vi "NI-DCPower Pulse Voltage Sequence T4.vi"() -> ()   [LabVIEW 2021, in "Main T4.lvlib"]
doc: "Demonstrates how to use the DCPower Pulse API to generate a Voltage Pulse Sequence. This example initializes a session, configures the Source Mode and the Output Function, configures the pulse parameters, initiates the pulse output sequence, and takes measurements."
uses:
  Main T4.lvlib
  DMM/controls/DMM Meas Type.ctl
  controls/Temp T4.ctl
  <instrlib>/niDCPower/nidcpower.llb/niDCPower Source Mode.ctl
  <instrlib>/niDCPower/nidcpower.llb/niDCPower Aperture Time Units.ctl
  <instrlib>/niDCPower/nidcpower.llb/niDCPower Output Function.ctl
  <instrlib>/niDCPower/nidcpower.llb/niDCPower Wait For Event - Event.ctl
  DMM/DMM T4.lvlib
panel:
  out "Cluster 2":T1={"Read?"=TRUE, "Temp"=0}
  in  "Cluster":T1={"Read?"=TRUE, "Temp"=0}
  in  "SMU DMM Measurement":T2
  in  "Pulse Current Limit Range":dbl=0.1 format="%#.6p"
  in  "Pulse Bias Voltage Level":dbl format="%.5p"
  in  "Pulse Voltage Level Range":dbl=6.0 format="%#.6p"
  in  "Pulse Current Limit":dbl=0.1 format="%.5p"
  in  "Pulse Bias Current Limit":dbl=0.1 format="%.5p"
  in  "Pulse Voltage Sequence":dbl[](array[numeric])=[1.0, 2.0, 3.0] format="%_6g"
  in  "Source Delays":dbl[](array[numeric])=[5e-05, 6e-05, 7e-05] format="%.3p"
  in  "Aperture Time (Sec)":dbl=0.0001
  out "Current Measurements":dbl[](array[numeric])
  out "Voltage Measurements":dbl[](array[numeric])
  in  "Pulse Bias Delay (Sec)":dbl=1e-06 format="%.3p"
  in  "Pulse Off Time (Sec)":dbl=0.005
  in  "Pulse On Time (Sec)":dbl=0.001
  in  "Load SMUs":refnum<k15>="Dev1" caption="Load SMU"
  in  "Load SMU Channel":string="0"
  # "Overview: This example outputs a sequence of voltage pulses and takes a voltage and current measurement at the peak of each pulse. \nRequirements: NI-DCPower\nInstructions:\n1. Select the appropriate device in the Resource Name control.\n2. Configure the pulse sequence that you would like to output.\n3. Run the VI."
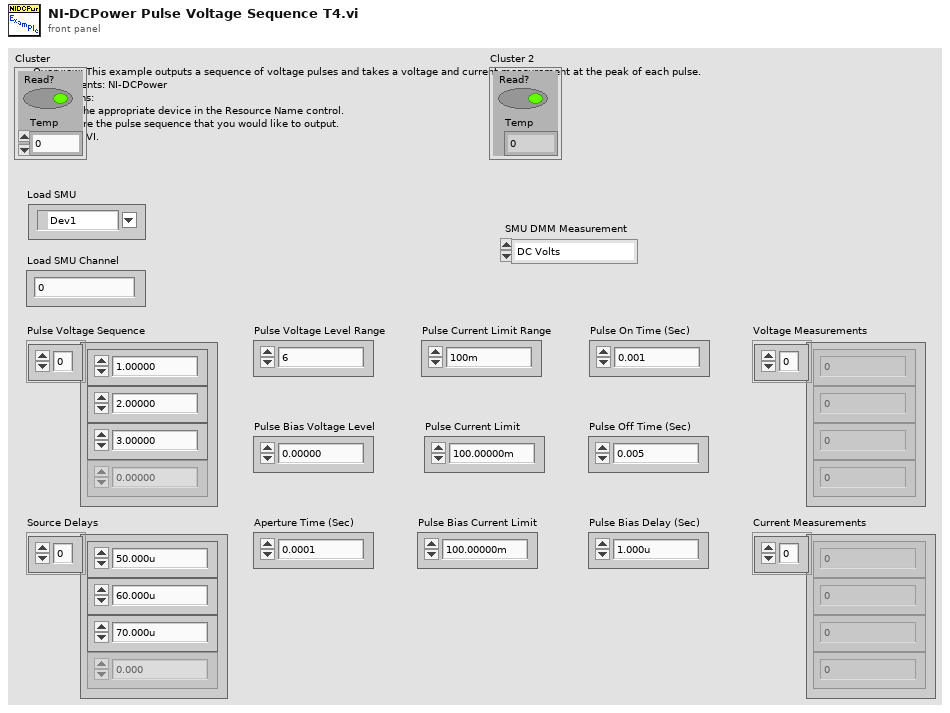
[diagram p1: front panel]
types:
  T1 = typedef "Temp T4.ctl" = cluster{"Read?":bool, "Temp":i32}
  T2 = typedef "DMM T4.lvlib/DMM Meas Type.ctl" = enum16{"DC Volts", "AC Volts", "DC Current", "AC Current", "2-wire Resistance", "4-wire Resistance", "Diode", "Frequency", "Period", "AC Volts DC Coupled", "Capacitance", "Inductance", "Temperature"}
  T3 = typedef "niDCPower Wait For Event - Event.ctl" = i32
  T4 = typedef "niDCPower Output Function.ctl" = i32
  T5 = typedef "niDCPower Aperture Time Units.ctl" = i32
  T6 = typedef "niDCPower Source Mode.ctl" = i32
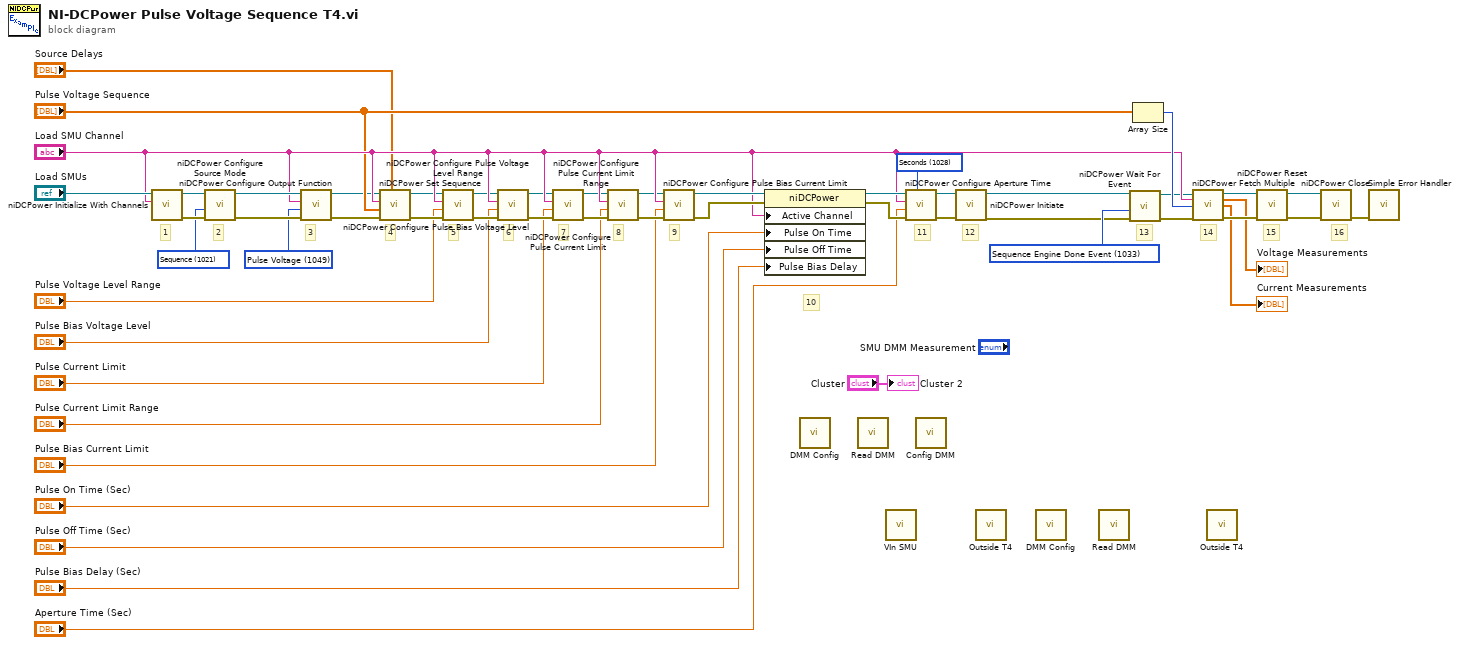
[diagram p0: block diagram]
diagram:
  w6 = T3 1033 items=["Source Complete Event"=1030, "Measure Complete Event"=1031, "Sequence Iteration Complete Event"=1032, "Sequence Engine Done Event"=1033, "Pulse Complete Event"=1051, "Ready For Pulse Trigger Event"=1052] ("event")
  w16 = T4 1049 items=["DC Voltage"=1006, "DC Current"=1007, "Pulse Voltage"=1049, "Pulse Current"=1050] ("output function")
  w29 = T5 1028 items=["Seconds"=1028, "Powerline Cycles"=1029] ("aperture time units")
  w48 = T6 1021 items=["Single Point"=1020, "Sequence"=1021] ("source mode")
  # "15"
  # "9"
  # "8"
  # "7"
  # "6"
  # "5"
  # "4"
  # "3"
  # "16"
  # "14"
  # "13"
  # "12"
  # "11"
  # "10"
  # "2"
  # "1"
  n1 = call <instrlib>:"niDCPower Initialize With Channels.vi"("channels"="Load SMU Channel", "resource name"="Load SMUs") -> ("error out"=w52:errorcluster, "instrument handle out"=w45:refnum<k15>)  [unwired: 3 in, 5 out]
  n2 = call <instrlib>:"niDCPower Configure Source Mode.vi"("error in (no error)"=w52, "source mode"=w48, "instrument handle"=w45) -> ("error out"=w46:errorcluster, "instrument handle out"=w47:refnum<k15>)  [unwired: 7 out]
  n3 = call <instrlib>:"niDCPower Configure Output Function.vi"("error in (no error)"=w46, "output function"=w16, "channel name"="Load SMU Channel", "instrument handle"=w47) -> ("error out"=w8:errorcluster, "instrument handle out"=w10:refnum<k15>)  [unwired: 6 out]
  n4 = call <instrlib>:"niDCPower Set Sequence.vi"("source delays"="Source Delays", "error in (no error)"=w8, "values"="Pulse Voltage Sequence", "channel name"="Load SMU Channel", "instrument handle"=w10) -> ("error out"=w25:errorcluster, "instrument handle out"=w9:refnum<k15>)  [unwired: 5 in]
  n5 = call <instrlib>:"niDCPower Configure Pulse Voltage Level Range.vi"("error in (no error)"=w25, "pulse voltage level range"="Pulse Voltage Level Range", "channel name"="Load SMU Channel", "instrument handle"=w9) -> ("error out"=w24:errorcluster, "instrument handle out"=w23:refnum<k15>)  [unwired: 6 in]
  n6 = call <instrlib>:"niDCPower Configure Pulse Bias Voltage Level.vi"("error in (no error)"=w24, "pulse bias voltage level"="Pulse Bias Voltage Level", "channel name"="Load SMU Channel", "instrument handle"=w23) -> ("error out"=w22:errorcluster, "instrument handle out"=w21:refnum<k15>)  [unwired: 6 in]
  n7 = call <instrlib>:"niDCPower Configure Pulse Current Limit.vi"("error in (no error)"=w22, "pulse current limit"="Pulse Current Limit", "channel name"="Load SMU Channel", "instrument handle"=w21) -> ("error out"=w20:errorcluster, "instrument handle out"=w19:refnum<k15>)  [unwired: 6 in]
  n8 = call <instrlib>:"niDCPower Configure Pulse Current Limit Range.vi"("error in (no error)"=w20, "pulse current limit range"="Pulse Current Limit Range", "channel name"="Load SMU Channel", "instrument handle"=w19) -> ("error out"=w18:errorcluster, "instrument handle out"=w17:refnum<k15>)  [unwired: 6 in]
  n9 = call <instrlib>:"niDCPower Configure Pulse Bias Current Limit.vi"("error in (no error)"=w18, "pulse bias current limit"="Pulse Bias Current Limit", "channel name"="Load SMU Channel", "instrument handle"=w17) -> ("error out"=w39:errorcluster, "instrument handle out"=w40:refnum<k15>)  [unwired: 6 in]
  n10 = property class="niDCPower"(reference=w40, error in=w39, "Active Channel"="Load SMU Channel", "Pulse On Time"="Pulse On Time (Sec)", "Pulse Off Time"="Pulse Off Time (Sec)", "Pulse Bias Delay"="Pulse Bias Delay (Sec)") -> (reference out=w31:refnum<k15>, error out=w33:errorcluster)
  n11 = call "DMM Config.vi"() -> ()  [unwired: 9 in, 3 out]
  n12 = call "Read DMM.vi"() -> ()  [unwired: 11 in, 1 out]
  n13 = call "VIn SMU.vi"() -> ()  [unwired: 9 in, 3 out]
  n14 = call <instrlib>:"niDCPower Configure Aperture Time.vi"("aperture time units"=w29, "error in (no error)"=w33, "aperture time"="Aperture Time (Sec)", "channel name"="Load SMU Channel", "instrument handle"=w31) -> ("error out"=w32:errorcluster, "instrument handle out"=w30:refnum<k15>)  [unwired: 5 in]
  n15 = call "Config DMM.vi"() -> ()  [unwired: 10 in, 2 out]
  n16 = call <instrlib>:"niDCPower Initiate.vi"("error in (no error)"=w32, "instrument handle"=w30) -> ("error out"=w2:errorcluster, "instrument handle out"=w3:refnum<k15>)  [unwired: 2 in, 6 out]
  n17 = call "Outside T4.vi"() -> ()  [unwired: 12 in]
  n18 = call "DMM Config.vi"() -> ()  [unwired: 9 in, 3 out]
  n19 = call "Read DMM.vi"() -> ()  [unwired: 11 in, 1 out]
  n20 = call <instrlib>:"niDCPower Wait For Event.vi"("error in (no error)"=w2, "event"=w6, "instrument handle"=w3) -> ("error out"=w4:errorcluster, "instrument handle out"=w5:refnum<k15>)  [unwired: 7 in]
  n21 = Array Size(array="Pulse Voltage Sequence") -> (size(s)=w34:i32)
  n22 = call <instrlib>:"niDCPower Fetch Multiple.vi"("instrument handle"=w5, "channel name"="Load SMU Channel", "count (1)"=w34, "error in (no error)"=w4) -> ("instrument handle out"=w36:refnum<k15>, "voltage measurements"=→"Voltage Measurements":dbl[], "current measurements"=→"Current Measurements":dbl[], "error out"=w51:errorcluster)  [unwired: 6 in, 2 out]
  n23 = call "Outside T4.vi"() -> ()  [unwired: 12 in]
  n24 = call <instrlib>:"niDCPower Reset.vi"("error in (no error)"=w51, "instrument handle"=w36) -> ("error out"=w43:errorcluster, "instrument handle out"=w42:refnum<k15>)  [unwired: 2 in, 6 out]
  n25 = call <instrlib>:"niDCPower Close.vi"("error in (no error)"=w43, "instrument handle"=w42) -> ("error out"=w44:errorcluster)  [unwired: 9 out]
  n26 = call <vilib>:"Simple Error Handler.vi"("error in (no error)"=w44) -> ()  [unwired: 1 in, 8 out]
  "Cluster 2" <- "Cluster"
